vi "SetParam.vi"(8 "error in (no error)":errorcluster caption="entrée d'erreur (pas d'erreur)", 10 "GroupShuffleSplit":T1={"n_splits"=5, "test_size"="0,2", "train_size"="None", "random_state"=-1} {"random_state" min=-1}, 11 "GroupShuffleSplit.lvclass":refnum<class "GroupShuffleSplit.lvclass">) -> (0 "error out":errorcluster caption="sortie d'erreur", 3 "GroupShuffleSplit.lvclass":refnum<class "GroupShuffleSplit.lvclass">)   [LabVIEW 2020, in "GroupShuffleSplit.lvclass"]
doc: "Set Parameters"
uses:
  GroupShuffleSplit.lvclass
  GroupShuffleSplit.lvclass/GroupShuffleSplit.ctl
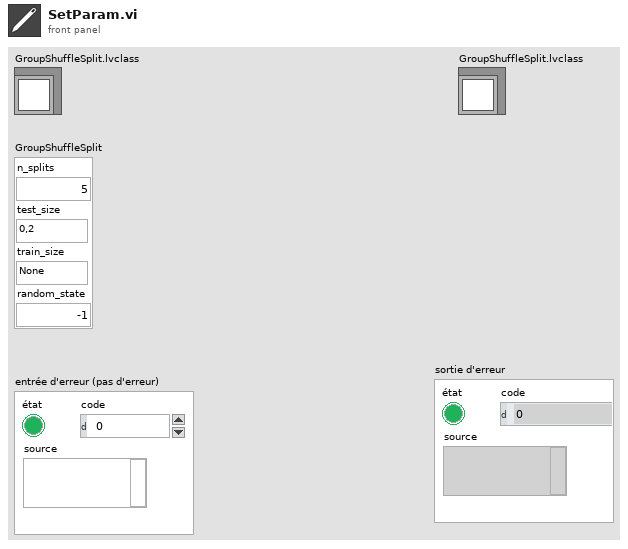
[diagram p1: front panel]
types:
  T1 = cluster{"n_splits":i32, "test_size":string, "train_size":string, "random_state":i32}
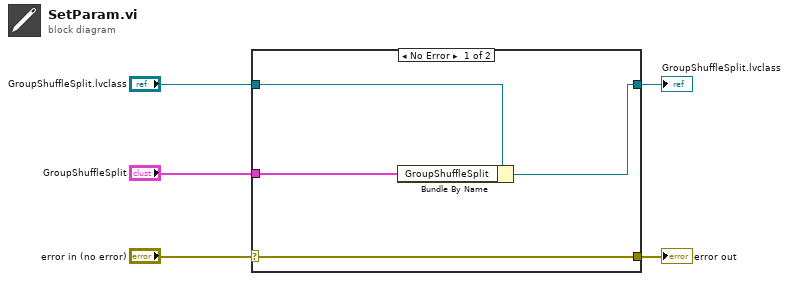
[diagram p0: block diagram]
diagram:
  n1 = case shown="No Error" "error in (no error)" {
    selector: "error in (no error)" -> [w9 w10]
    tunnel: [w9 w10] -> w4
    tunnel: [w7 w11] -> w2
    tunnel: "GroupShuffleSplit.lvclass" -> [w8 w11]
    tunnel: "GroupShuffleSplit" -> [w6 _]
    frame No Error {
      n2 = Bundle By Name(cluster=w8, "GroupShuffleSplit"=w6) -> (w7:refnum<class "GroupShuffleSplit.lvclass">)
    }
    frame Error {
    }
  }
  "error out" <- w4
  "GroupShuffleSplit.lvclass" <- w2
